vi "Lab1.vi"() -> ()   [LabVIEW 2014]
uses:
  <vilib>/Instr/_visa.llb/VISA Configure Serial Port (Instr).vi
  <vilib>/Utility/file.llb/Read From Spreadsheet File (DBL).vi
  <vilib>/imath/engines/lvmath2/RunTimeEngine/NodeEndStatement/NIMS_NodeEndStatement_Output.vi
  <instcachedir>/0/NIMS_NodeEndStatement_Output_53EC0D466D134D7ABD903AC30B43404B.lvgen/NIMS_NodeEndStatement_Output_53EC0D466D134D7ABD903AC30B43404B_001.vi
  <vilib>/imath/engines/lvmath2/RunTimeEngine/ErrorHandling/NIMS_Finalize Error.vi
  <vilib>/Utility/file.llb/Write To Spreadsheet File (DBL).vi
panel:
  in  "Calculate transformation":bool
  in  "delete":bool
  in  "input path for new points":path
  out "New point list":dbl[][](array[numeric])
  in  "Array":dbl[][](array[numeric])
  out "New point global":dbl[](array[numeric])
  out "Answer 2":string
  in  "Timeout [ms] 2":u32=5000
  in  "Request 2":string
  in  "Stop everything 2":bool
  in  "Send request 2":bool
  out "resY":dbl[](array[numeric])
  out "resX":dbl[](array[numeric])
  in  "File path for global coordinates":path
  out "Global coordinates":dbl[][](array[numeric]) format="%0.3f"
  out "Local coordinates":dbl[][](array[numeric])
  out "Local coordinates measurement":dbl[][](array[numeric])
  in  "Delete row":i32
  in  "Timeout [ms]":u32=5000
  in  "Stop everything":bool
  in  "Send request":bool
  out "Answer":string
  in  "Request":string
  in  "parity (0:none)":enum16{"None", "Odd", "Even", "Mark", "Space"}(ring)
  in  "data bits (8)":u16=8 min=5 max=8 step=1
  in  "baud rate (9600)":u32=9600
  in  "VISA resource name":refnum<visa-resource-name>
  # "Measure Local Coordinates of Known Points"
  # "Measure new Points in Global Reference System"
  # "Calculate Helmert Transformation"
  # "Steering of Tachymeter"
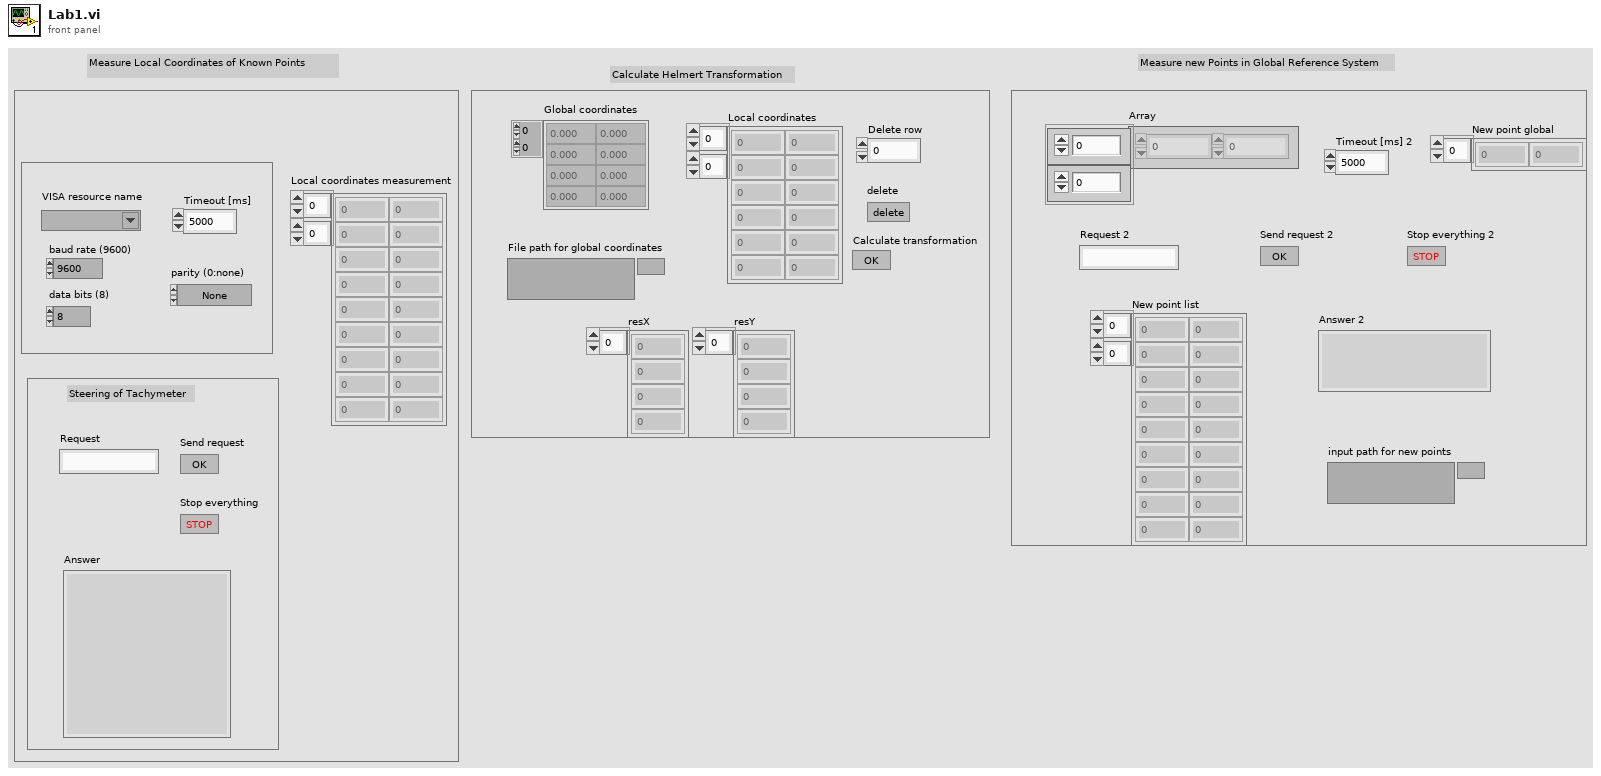
[diagram p1: front panel]
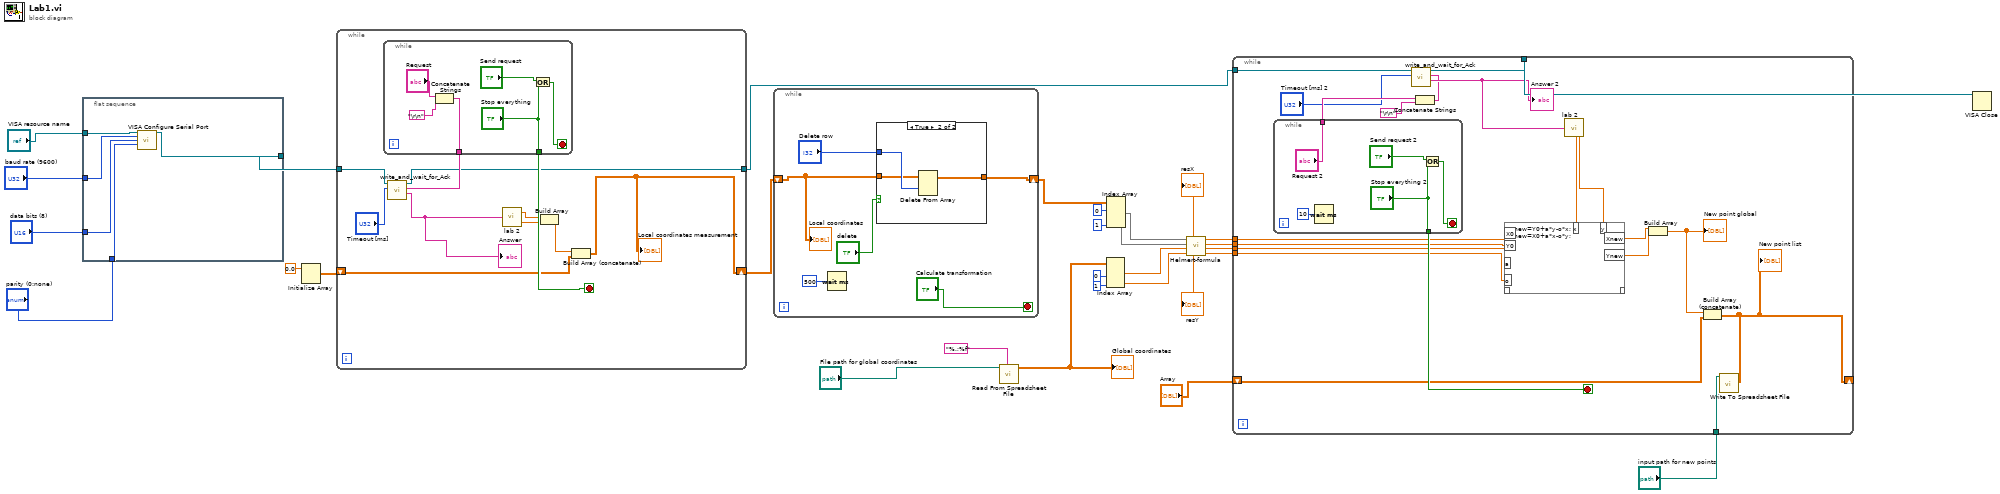
[diagram p0: block diagram]
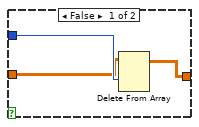
[diagram p2: hidden frame]
diagram:
  n1 = flat-sequence {
    tunnel: "VISA resource name" -> [w35]
    tunnel: "parity (0:none)" -> [w34]
    tunnel: "data bits (8)" -> [w33]
    tunnel: "baud rate (9600)" -> [w32]
    tunnel: [w31] -> w26
    frame #0 {
      n2 = call-poly "VISA Configure Serial Port"("VISA resource name"=w35, "baud rate (9600)"=w32, "data bits (8)"=w33, "parity (0:none)"=w34) -> ("VISA resource name out"=w31:refnum<visa-resource-name>)  [unwired: 10 in, 1 out]
    }
  }
  n3 = Initialize Array(0.0 ("element")) -> (w1:dbl[][])  [unwired: 2 in]
  n4 = while {
    tunnel: w26 -> [w41]
    tunnel: [w36] -> w10
    shift-right: [w44] -> w2
    shift-left: w1 -> [w43]
    stop <- w46 stop-if-true
    n5 = while {
      tunnel: [w50] -> w42
      tunnel: ["Stop everything"] -> w46
      stop <- w47 stop-if-true
      n6 = Concatenate Strings("Request", "\r\n") -> (w50:string)
      n7 = Or(x="Send request", y="Stop everything") -> (x .or. y?=w47:bool)
    }
    n8 = call "write_and_wait_for_Ack.vi"("request"=w42, "Timeout [ms]"="Timeout [ms]", "VISA resource name"=w41) -> ("result"=w39:string, "VISA resource name out"=w36:refnum<visa-resource-name>)  [unwired: 4 in, 1 out]
    "Answer" <- w39
    n9 = call "lab 2.vi"("String Input"=w39) -> ("Hz"=w38:dbl, "V"=w37:dbl)
    n10 = Build Array(w38, w37) -> (w45:dbl[])
    n11 = Build Array (concatenate)(w45, w43) -> (w44:dbl[][])
    "Local coordinates measurement" <- w44
  }
  n12 = while {
    shift-right: [w54] -> w3
    shift-left: w2 -> [w53]
    stop <- "Calculate transformation" stop-if-true
    n13 = Wait (ms)(milliseconds to wait=u32 500) -> ()  [unwired: 1 out]
    n14 = case shown="True" "delete" {
      tunnel: "Delete row" -> [w61 w64]
      tunnel: w53 -> [w60 w63]
      tunnel: [w59 w62] -> w54
      frame False {
        n15 = Delete From Array(array=w60, index (row)=w61) -> (array with subset deleted=w59:dbl[][])  [unwired: 2 in, 1 out]
      }
      frame True {
        n16 = Delete From Array(array=w63, index (row)=w64) -> (array with subset deleted=w62:dbl[][])  [unwired: 2 in, 1 out]
      }
    }
    "Local coordinates" <- w53
  }
  n17 = call-poly <vilib>:"Read From Spreadsheet File.vi"("format (%.3f)"="%.;%f", "file path (dialog if empty)"="File path for global coordinates") -> ("all rows"=w20:dbl[][])  [unwired: 5 in, 4 out]
  "Global coordinates" <- w20
  n18 = Index Array(array=w20, index (col) #1=0 ("disabled index (col)"), index (col) #2=1 ("index (col)")) -> (element #1=w15:dbl[], element #2=w14:dbl[])  [unwired: 2 in]
  n19 = Index Array(array=w3, index (row) #1=0 ("index (row)"), index (col) #2=1 ("disabled index (col)")) -> (element #1=w17:dbl[], element #2=w16:dbl[])  [unwired: 2 in]
  n20 = call "Helmert-formula.vi"("Y"=w14, "X"=w15, "y"=w16, "x"=w17) -> ("o"=w6:dbl, "a"=w7:dbl, "Y0"=w8:dbl, "X0"=w9:dbl, "resY"=→"resY":dbl[], "resX"=→"resX":dbl[])  [unwired: 2 in]
  n21 = while {
    tunnel: [w67] -> w11
    tunnel: w10 -> [w68]
    tunnel: w9 -> [w79]
    tunnel: w8 -> [w78]
    tunnel: w7 -> [w77]
    tunnel: w6 -> [w76]
    tunnel: "input path for new points" -> [w72]
    shift-right: [w70] -> _
    shift-left: "Array" -> [w71]
    stop <- w82 stop-if-true
    n22 = while {
      tunnel: ["Stop everything 2"] -> w82
      tunnel: ["Request 2"] -> w83
      stop <- w135 stop-if-true
      n23 = Wait (ms)(milliseconds to wait=u32 10) -> ()  [unwired: 1 out]
      n24 = Or(x="Send request 2", y="Stop everything 2") -> (x .or. y?=w135:bool)
    }
    n25 = Concatenate Strings(w83, "\r\n") -> (w65:string)
    n26 = call "write_and_wait_for_Ack.vi"("request"=w65, "Timeout [ms]"="Timeout [ms] 2", "VISA resource name"=w68) -> ("result"=w66:string, "VISA resource name out"=w67:refnum<visa-resource-name>)  [unwired: 4 in, 1 out]
    "Answer 2" <- w66
    n27 = call "lab 2.vi"("String Input"=w66) -> ("Hz"=w81:dbl, "V"=w80:dbl)
    n28 = mathscript code="Ynew=Y0+a*y-o*x;\nXnew=X0+a*x-o*y;"("X0"=w79, "Y0"=w78, "a"=w77, "o"=w76, "x"=w80, "y"=w81) -> ("Xnew"=w75:dbl, "Ynew"=w74:dbl)  [unwired: 1 in, 1 out]
    n29 = Build Array(w75, w74) -> (w73:dbl[])
    "New point global" <- w73
    n30 = Build Array (concatenate)(w73, w71) -> (w70:dbl[][])
    "New point list" <- w70
    n31 = call-poly <vilib>:"Write To Spreadsheet File.vi"("2D data"=w70, "file path (dialog if empty)"=w72) -> ()  [unwired: 6 in, 1 out]
  }
  n32 = VISA Close(VISA resource name=w11) -> ()  [unwired: 1 in, 1 out]
